vi "SM motor repeat tw.vi"(7 "Waiting time (s)":dbl=3.0, 8 "Stop motor":bool, 9 "Move":bool, 10 "SM setting":T1={"Acceleration (mm/sec^2)"=1000.0, "Velocity (mm/sec)"=1.0, "Position (mm)"=0.0} {"Position (mm)" format="%.3f"; "Velocity (mm/sec)" format="%.3f"; "Acceleration (mm/sec^2)" format="%.3f"}, 11 "SM Config":T2={"VISA Serial ref"="COM3", "Motor Config"={"DriveRatio (mm/rev)"=10.16, "PosLimit + (mm)"=200.0, "PosLimit - (mm)"=0.0, "EncoderRatio (count/rev)"=2000.0, "MotorType"=enum."SM17"}} {"Motor Config"."EncoderRatio (count/rev)" format="%.2f"; "Motor Config"."PosLimit - (mm)" format="%.3f"; "Motor Config"."PosLimit + (mm)" format="%.3f"; "Motor Config"."DriveRatio (mm/rev)" format="%.2f"}) -> (2 "Position (mm)":dbl)   [LabVIEW 2015]
uses:
  magnetometers/smi/labview/CPM20Software/SmartMotor.llb/SM Config.ctl
  magnetometers/smi/labview/CPM20Software/SmartMotor.llb/SM MotorConfig.ctl
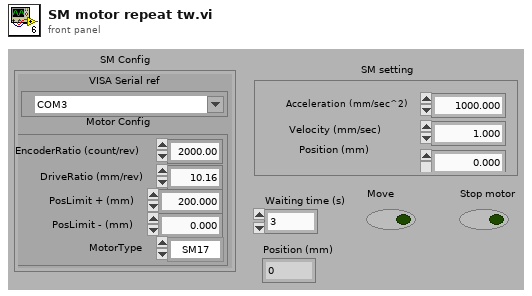
[diagram p1: front panel]
types:
  T1 = cluster{"Acceleration (mm/sec^2)":dbl, "Velocity (mm/sec)":dbl, "Position (mm)":dbl}
  T2 = typedef "SM Config.ctl" = cluster{"VISA Serial ref":refnum<visa-resource-name>, "Motor Config":T3}
  T3 = typedef "SM MotorConfig.ctl" = cluster{"DriveRatio (mm/rev)":dbl, "PosLimit + (mm)":dbl, "PosLimit - (mm)":dbl, "EncoderRatio (count/rev)":dbl, "MotorType":enum16{"SM17", "SM23", "SM34", "SM42", "SM56"}}
  T4 = cluster{"Acceleration (mm/sec^2)":dbl, "Velocity (mm/sec)":dbl, "PosLimit - (mm)":dbl}
  T5 = typedef "SM Status.ctl" = cluster{"Trajectory In Progress":bool, "(+) Pos Limit":bool, "(-) Pos Limit":bool, "Index Report Available":bool, "Wraparound":bool, "Position Error":bool, "Excessive Temp":bool, "Motor off":bool}
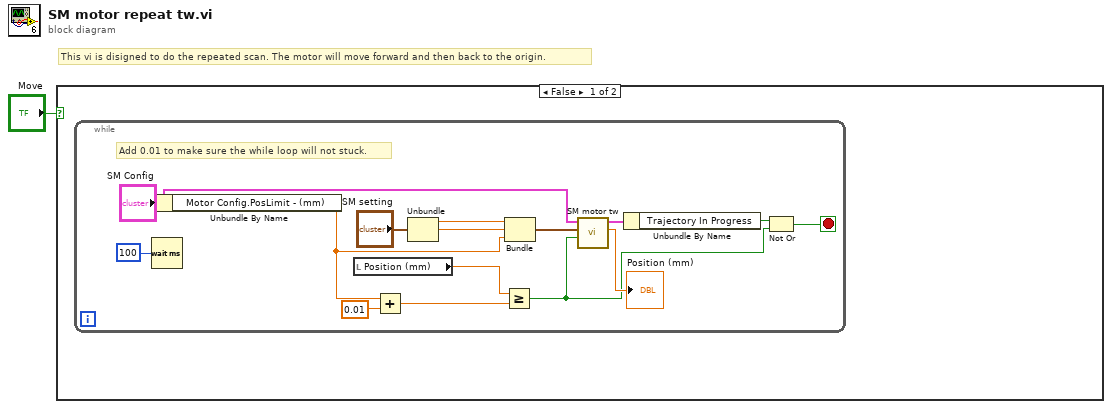
[diagram p0: block diagram]
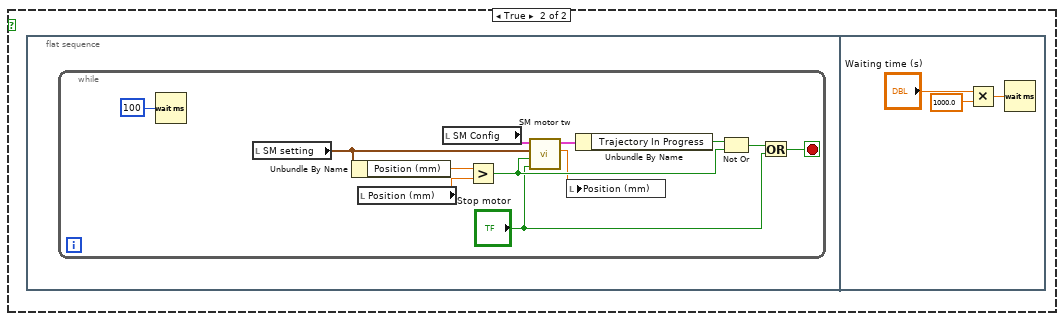
[diagram p2: hidden frame]
diagram:
  # "This vi is disigned to do the repeated scan. The motor will move forward and then back to the origin."
  n1 = case shown="False" "Move" {
    frame False {
      n2 = while {
        stop <- w10 stop-if-true
        # "Add 0.01 to make sure the while loop will not stuck."
        n3 = Wait (ms)(milliseconds to wait=u32 100) -> ()  [unwired: 1 out]
        n4 = Unbundle By Name("SM Config") -> ("Motor Config.PosLimit - (mm)"=w5:dbl)
        n5 = local read "Position (mm)"() -> (w7:dbl)
        n6 = Add(x=w5, y=0.01) -> (x+y=w6:dbl)
        n7 = Unbundle("SM setting") -> ("Acceleration (mm/sec^2)"=w14:dbl, "Velocity (mm/sec)"=w13:dbl)  [unwired: 1 out]
        n8 = Greater Or Equal?(x=w7, y=w6) -> (x >= y?=w8:bool)
        n9 = Bundle("Acceleration (mm/sec^2)"=w14, "Velocity (mm/sec)"=w13, "PosLimit - (mm)"=w5) -> (w12:T4)  [unwired: 1 out]
        n10 = call "SM motor tw.vi"("SM Config"="SM Config", "SM setting"=w12, "Move"=w8) -> ("Status"=w11:T5, "Position (mm)"=→"Position (mm)":dbl)  [unwired: 1 in, 5 out]
        n11 = Unbundle By Name(w11) -> ("Trajectory In Progress"=w9:bool)
        n12 = Not Or(1:w8, 2:w9) -> (0:w10:bool)
      }
    }
    frame True {
      n13 = flat-sequence {
        frame #0 {
          n14 = while {
            stop <- w20 stop-if-true
            n15 = Wait (ms)(milliseconds to wait=u32 100) -> ()  [unwired: 1 out]
            n16 = local read "SM setting"() -> (w23:T1)
            n17 = Unbundle By Name(w23) -> ("Position (mm)"=w22:dbl)
            n18 = local read "Position (mm)"() -> (w17:dbl)
            n19 = local read "SM Config"() -> (w25:T2)
            n20 = Greater?(x=w22, y=w17) -> (0:w26:bool)
            n21 = call "SM motor tw.vi"("SM Config"=w25, "SM setting"=w23, "Move"=w26, "Stop motion"="Stop motor") -> ("Status"=w27:T5, "Position (mm)"=w24:dbl)  [unwired: 5 out]
            n22 = local write "Position (mm)"(w24) -> ()
            n23 = Unbundle By Name(w27) -> ("Trajectory In Progress"=w21:bool)
            n24 = Not Or(1:w26, 2:w21) -> (0:w19:bool)
            n25 = Or(x=w19, y="Stop motor") -> (x .or. y?=w20:bool)
          }
        }
        frame #1 {
          n26 = Multiply(x="Waiting time (s)", y=1000.0) -> (x*y=w29:dbl)
          n27 = Wait (ms)(milliseconds to wait=w29) -> ()  [unwired: 1 out]
        }
      }
    }
  }
